vi "Teleop - Apply Speed Reduction.vi"(4 "Gain":dbl, 6 "Reduce Speed":bool, 8 "In 2":dbl, 11 "In 1":dbl) -> (0 "Out 2":dbl, 3 "Out1":dbl)   [LabVIEW 2015]
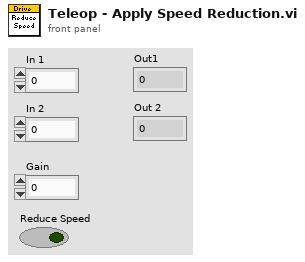
[diagram p1: front panel]
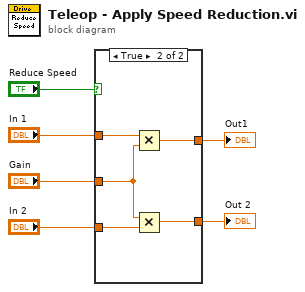
[diagram p0: block diagram]
diagram:
  n1 = case shown="True" "Reduce Speed" {
    tunnel: "Gain" -> [_ w13]
    tunnel: "In 1" -> [w8 w12]
    tunnel: "In 2" -> [w7 w11]
    tunnel: [w8 w10] -> w1
    tunnel: [w7 w9] -> w2
    frame False {
    }
    frame True {
      n2 = Multiply(x=w12, y=w13) -> (x*y=w10:dbl)
      n3 = Multiply(x=w13, y=w11) -> (x*y=w9:dbl)
    }
  }
  "Out1" <- w1
  "Out 2" <- w2
